vi "Detect Controller.vi"(6 "Network Adapters":bool caption="Network Adapters (F)", 8 "error in":errorcluster, 11 "Controller in":refnum<class "Controller.lvclass">) -> (0 "error out":errorcluster, 3 "Controller out":refnum<class "Controller.lvclass">)   [LabVIEW 2016, in "SMI.lvlib" / "Controller.lvclass"]
uses:
  Controller.lvclass
  C:/GitHub/SystemManagementAndInformation/source/classes/SysCfg Device/SysCfg Device.lvclass
  C:/GitHub/SystemManagementAndInformation/source/classes/Device/Device.lvclass
  SysCfg Device/SysCfg Device.lvclass/SysCfg Device.ctl
  Device/Device.lvclass/Device.ctl
  Controller.lvclass/Controller.ctl
  SysCfg Device/Accessor Methods/Read SysCfg Session.vi
  SysCfg Device/Accessor Methods/Write SysCfg Session.vi
  Device/Accessor Methods/Write Vendor Name.vi
  Device/Accessor Methods/Write Product Name.vi
  Device/Accessor Methods/Write Product ID.vi
  Device/Accessor Methods/Write Serial Number.vi
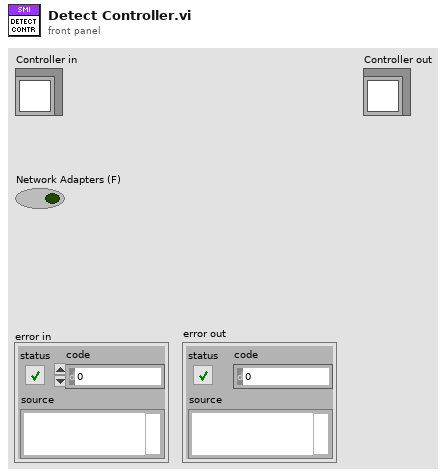
[diagram p1: front panel]
types:
  T1 = typedef "SMI.lvlib/Controller.lvclass/ControllerInformation.ctl" = cluster{"SysCfg Session":refnum<data-value>, "System Hardware Reference":refnum<data-value>, "Vendor Name":string, "Product Name":string, "Product ID":u16, "Serial Number":string, "Device Information":T2, "Primary Network Adapter":T3, "Secondary Network Adapters":T3[]}
  T2 = typedef "SMI.lvlib/Controller.lvclass/DeviceInformation.ctl" = cluster{"Resource":string, "Device Class":string, "System Start Time":timestamp, "Current Time":timestamp, "Time Zone":string, "Firmware Revision":string, "Image Title":string, "Image Version":string, "System Status":string}
  T3 = typedef "SMI.lvlib/Controller.lvclass/NetworkAdapterSettings.ctl" = cluster{"IP Address":string, "MAC Address":string, "IP Address Request Mode":u32, "SubnetMask":string, "Gateway":string, "DNS Server":string, "Adapter Mode":u32, "Adapter Type":u32}
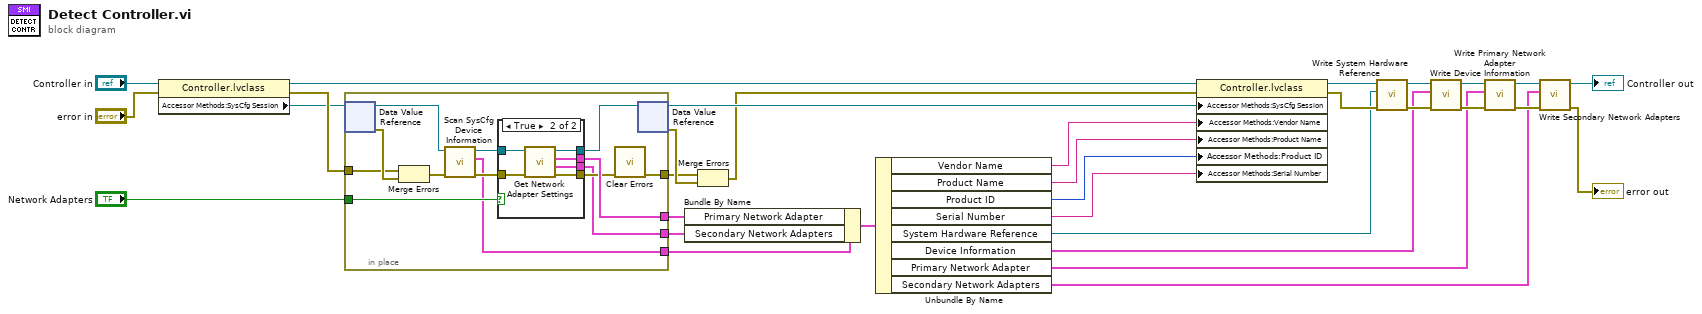
[diagram p0: block diagram]
diagram:
  n1 = property class="Controller.lvclass"(reference="Controller in", error in="error in") -> (reference out=w8:refnum<class "Controller.lvclass">, error out=w26:errorcluster, "Accessor Methods:SysCfg Session"=w7:refnum<data-value>)
  n2 = in-place {
    in-place-border: "Network Adapters" -> [w45]
    in-place-border: [w42] -> w31
    in-place-border: [w40] -> w30
    in-place-border: [w39] -> w29
    in-place-border: w26 -> [w35]
    in-place-border: [w38] -> w5
    n3 = in-place-dvr #1(w7) -> (w37:refnum<k21>, w36:errorcluster)
    n4 = Merge Errors(w35, w36) -> (w34:errorcluster)
    n5 = call "Scan SysCfg Device Information.vi"("error in"=w34, "Refnum in"=w37) -> ("error out"=w43:errorcluster, "Network Device"=w40:T1, "Refnum out"=w44:refnum<k21>)  [unwired: 7 in]
    n6 = case shown="True" w45 {
      tunnel: w44 -> [w47 w53]
      tunnel: w43 -> [w46 w52]
      tunnel: [_ w51] -> w42
      tunnel: [w47 w50] -> w33
      tunnel: [w46 w49] -> w41
      tunnel: [_ w48] -> w39
      frame False {
      }
      frame True {
        n7 = call "Get Network Adapter Settings.vi"("error in"=w52, "Refnum in"=w53) -> ("error out"=w49:errorcluster, "Secondary Network Adapters"=w48:T3[], "Primary Network Adapter"=w51:T3, "Refnum out"=w50:refnum<k21>)  [unwired: 6 in]
      }
    }
    n8 = call <vilib>:"Clear Errors.vi"("error in (no error)"=w41) -> ("error out"=w38:errorcluster)  [unwired: 5 in, 1 out]
    n9 = in-place-dvr #1(w33) -> (w3:refnum<data-value>, w6:errorcluster)
  }
  n10 = Bundle By Name(cluster=w30, "Primary Network Adapter"=w31, "Secondary Network Adapters"=w29) -> (w25:T1)
  n11 = Merge Errors(w5, w6) -> (w1:errorcluster)
  n12 = Unbundle By Name(w25) -> ("Vendor Name"=w4:string, "Product Name"=w11:string, "Product ID"=w10:u16, "Serial Number"=w9:string, "System Hardware Reference"=w2:refnum<data-value>, "Device Information"=w16:T2, "Primary Network Adapter"=w15:T3, "Secondary Network Adapters"=w14:T3[])
  n13 = property class="Controller.lvclass"(reference=w8, error in=w1, "Accessor Methods:SysCfg Session"=w3, "Accessor Methods:Vendor Name"=w4, "Accessor Methods:Product Name"=w11, "Accessor Methods:Product ID"=w10, "Accessor Methods:Serial Number"=w9) -> (reference out=w13:refnum<class "Controller.lvclass">, error out=w12:errorcluster)
  n14 = call "Write System Hardware Reference.vi"("error in"=w12, "System Hardware Reference"=w2, "Controller in"=w13) -> ("error out"=w20:errorcluster, "Controller out"=w21:refnum<class "Controller.lvclass">)  [unwired: 7 in]
  n15 = call "Write Device Information.vi"("error in (no error)"=w20, "Device Information"=w16, "Controller in"=w21) -> ("error out"=w19:errorcluster, "Controller out"=w22:refnum<class "Controller.lvclass">)  [unwired: 7 in]
  n16 = call "Write Primary Network Adapter.vi"("error in (no error)"=w19, "Network Adapter Settings"=w15, "Controller in"=w22) -> ("error out"=w23:errorcluster, "Controller out"=w24:refnum<class "Controller.lvclass">)  [unwired: 7 in]
  n17 = call "Write Secondary Network Adapters.vi"("error in (no error)"=w23, "Secondary Network Adapters"=w14, "Controller in"=w24) -> ("error out"=→"error out":errorcluster, "Controller out"=→"Controller out":refnum<class "Controller.lvclass">)  [unwired: 7 in]
